vi "GetOpStateTags.vi"(10 "tags":T1[](array[typedef]), 11 "data group":string) -> (2 "op state tag id":string)   [LabVIEW 2017, in "OpState.lvlib"]
uses:
  <vilib>/addons/InsightCM/Devices/Shared/Common/OpState/OpState.lvlib
  <vilib>/addons/InsightCM/MessageBus/Base/controls/Tag.ctl
  <vilib>/addons/InsightCM/MessageBus/Base/controls/KeyValuePair.ctl
  <vilib>/addons/InsightCM/Utilities/DeviceModelHelpers/DeviceModelHelpers.lvlib
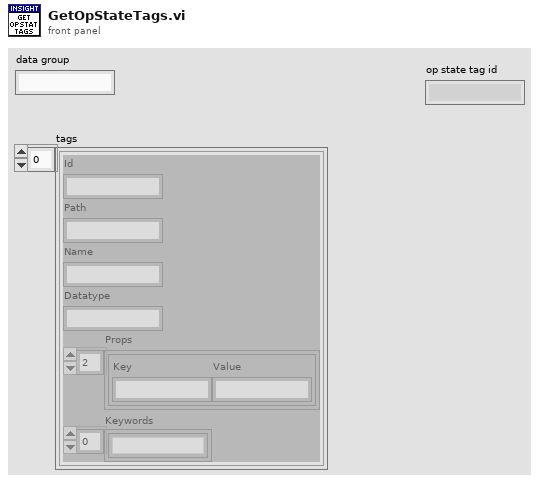
[diagram p1: front panel]
types:
  T1 = typedef "Tag.ctl" = cluster{"Id":string, "Path":string, "Name":string, "Datatype":string, "Props":T2[], "Keywords":string[]}
  T2 = typedef "KeyValuePair.ctl" = cluster{"Key":string, "Value":string}
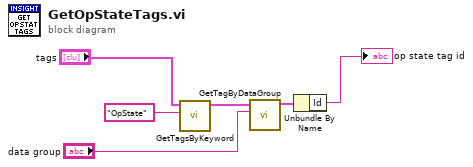
[diagram p0: block diagram]
diagram:
  n1 = call <vilib>:"GetTagsByKeyword.vi"("keyword"="OpState", "tags"="tags") -> ("matches"=w5:T1[])  [unwired: 9 in]
  n2 = call <vilib>:"GetTagByDataGroup.vi"("data group"="data group", "matches"=w5) -> ("Tag"=w3:T1)  [unwired: 8 in, 1 out]
  n3 = Unbundle By Name(w3) -> ("Id"=→"op state tag id":string)
